vi "source_read_voltage.vi"(8 "error in (no error)":errorcluster, 11 "VISA resource name":refnum<visa-resource-name>) -> (0 "error out":errorcluster, 2 "Value":sgl, 3 "VISA resource name out":refnum<visa-resource-name>)   [LabVIEW 2020]
doc: "Reads current voltage measured by source meter."
panel:
  out "return count 0":u32
  out "return count 1":u32
  out "read buffer":string
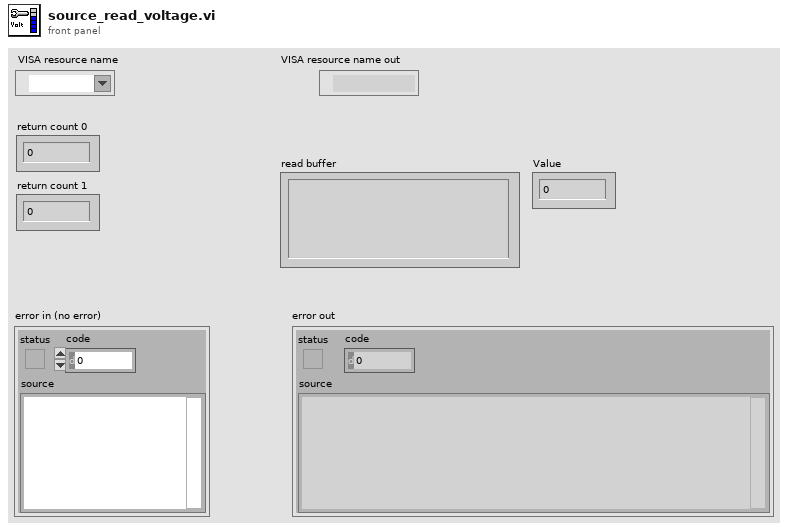
[diagram p1: front panel]
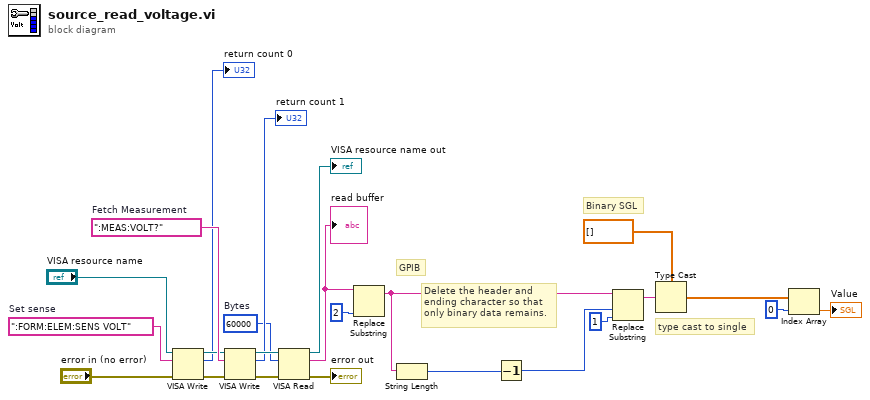
[diagram p0: block diagram]
diagram:
  w6 = ":FORM:ELEM:SENS VOLT"  # Set sense
  w24 = ":MEAS:VOLT?"  # Fetch Measurement
  w18 = u32 60000  # Bytes
  # "Binary SGL"
  # "Delete the header and ending character so that only binary data remains."
  # "GPIB"
  # "type cast to single"
  n1 = VISA Write(VISA resource name="VISA resource name", write buffer=w6, error in (no error)="error in (no error)") -> (VISA resource name out=w4:refnum<visa-resource-name>, return count=→"return count 0":u32, error out=w2:errorcluster)
  n2 = VISA Write(VISA resource name=w4, write buffer=w24, error in (no error)=w2) -> (VISA resource name out=w21:refnum<visa-resource-name>, return count=→"return count 1":u32, error out=w20:errorcluster)
  n3 = VISA Read(VISA resource name=w21, byte count=w18, error in (no error)=w20) -> (VISA resource name out=→"VISA resource name out":refnum<visa-resource-name>, read buffer=w8:string, error out=→"error out":errorcluster)  [unwired: 1 out]
  "read buffer" <- w8
  n4 = Replace Substring(2:2 ("length (len. of substring)"), 5:w8) -> (1:w16:string)  [unwired: 2 in, 1 out]
  n5 = String Length(string=w16) -> (length=w15:i32)
  n6 = Decrement(x=w15) -> (x-1=w14:i32)
  n7 = Replace Substring(2:1 ("length (len. of substring)"), 3:w14, 5:w16) -> (1:w11:string)  [unwired: 1 in, 1 out]
  n8 = Type Cast(type=sgl[] [], x=w11) -> (*(type *) &x=w10:sgl[])
  n9 = Index Array(array=w10, index=0) -> (element=→"Value":sgl)
